vi "Get Visible.vi"(7 "Hide if children are hidden? [T]":bool=TRUE, 8 "error in (no error)":errorcluster, 11 "IContainer in":refnum<class "IContainer.lvclass">) -> (0 "error out":errorcluster, 2 "Visible?":bool, 3 "IContainer out":refnum<class "IContainer.lvclass">, 4 "Item visible?":bool)   [LabVIEW 2013, in "IContainer.lvclass"]
doc: "Copyright 2018, Wiebe Walstra, wiebe@carya.nl."
uses:
  IContainer.lvclass
  IObject.lvclass
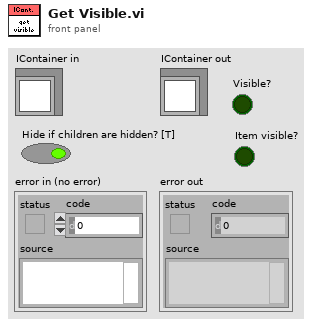
[diagram p1: front panel]
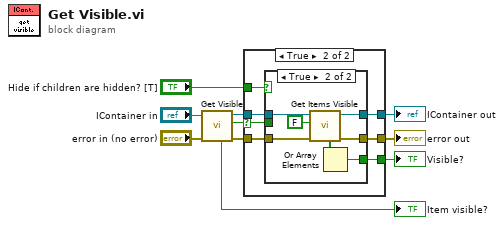
[diagram p0: block diagram]
diagram:
  n1 = call-parent "Get Visible.vi"("error in (no error)"="error in (no error)", "IObject in"="IContainer in") -> ("error out"=w5:errorcluster, "Visible?"=w3:bool, "IObject out"=w7:refnum<class "IContainer.lvclass">, "Item visible?"=→"Item visible?":bool)  [unwired: 6 in]
  n2 = case shown="True" w3 {
    selector: w3 -> [w13 w15]
    tunnel: w7 -> [w12 w20]
    tunnel: [w12 w19] -> w6
    tunnel: w5 -> [w11 w18]
    tunnel: [w11 w17] -> w4
    tunnel: [w13 w16] -> w2
    tunnel: "Hide if children are hidden? [T]" -> [_ w14]
    frame False {
    }
    frame True {
      n3 = case shown="True" w14 {
        tunnel: w20 -> [w22 w30]
        tunnel: [w22 w29] -> w19
        tunnel: w18 -> [w21 w28]
        tunnel: [w21 w27] -> w17
        tunnel: [w23 w24] -> w16
        tunnel: w15 -> [w23 _]
        frame False {
        }
        frame True {
          n4 = call "Get Items Visible.vi"("error in (no error)"=w28, "Return all? [T]"=FALSE, "IContainer in"=w30) -> ("error out"=w27:errorcluster, "IContainer out"=w29:refnum<class "IContainer.lvclass">, "Items visible"=w25:bool[])  [unwired: 5 in, 1 out]
          n5 = Or Array Elements(Boolean array=w25) -> (logical OR=w24:bool)
        }
      }
    }
  }
  "error out" <- w4
  "IContainer out" <- w6
  "Visible?" <- w2
